vi "calcMotorTemperature.vi"(8 "error in (no error)":errorcluster, 11 "Thermocouple in":refnum<class "Thermocouple.lvclass">) -> (0 "error out":errorcluster, 3 "Thermocouple out":refnum<class "Thermocouple.lvclass">)   [LabVIEW 2013, in "Thermocouple.lvclass"]
uses:
  Thermocouple.lvclass
  Thermocouple.lvclass/Thermocouple.ctl
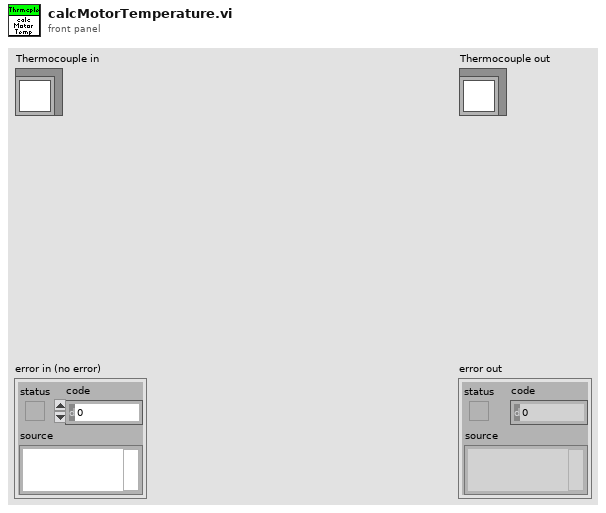
[diagram p1: front panel]
types:
  T1 = typedef "MotorOverheatTemperature.ctl" = dbl[unit]
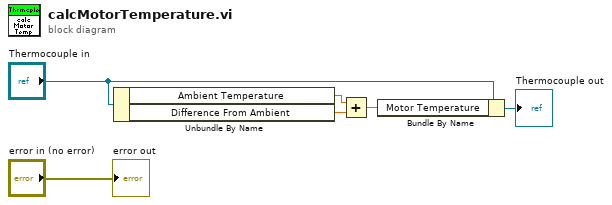
[diagram p0: block diagram]
diagram:
  n1 = Unbundle By Name("Thermocouple in") -> ("Ambient Temperature"=w5:T1, "Difference From Ambient"=w4:dbl[unit])
  n2 = Add(x=w5, y=w4) -> (x+y=w3:T1)
  n3 = Bundle By Name(cluster="Thermocouple in", "Motor Temperature"=w3) -> (→"Thermocouple out":refnum<class "Thermocouple.lvclass">)
  "error out" <- "error in (no error)"
